vi "ForLoop_AutoIndexing.vi"() -> ()   [LabVIEW 2019]
panel:
  out "Numeric":dbl
  in  "Array":dbl[](array[numeric])
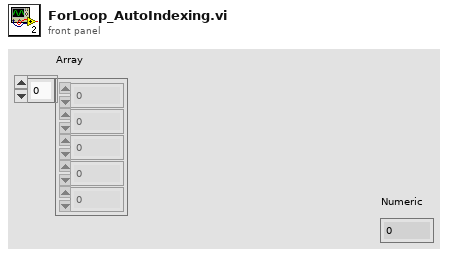
[diagram p1: front panel]
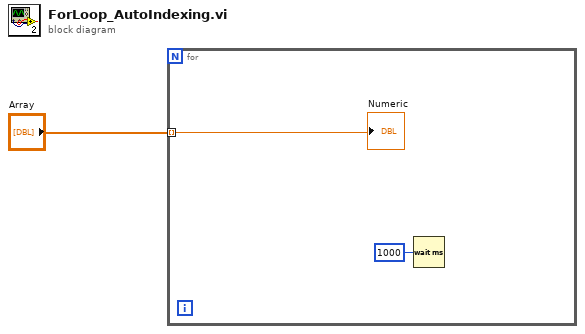
[diagram p0: block diagram]
diagram:
  n1 = for {
    tunnel: "Array" -> [w3] mode=indexing
    n2 = Wait (ms)(milliseconds to wait=u32 1000) -> ()  [unwired: 1 out]
    "Numeric" <- w3
  }
